vi "FlatToRichw4lvgrpc_Msg_ToClient_3.vi"(5 "OutputClusterType":T1, 11 "InputCluster":T3) -> (3 "OutputCluster":T1)   [LabVIEW 2019, in "Generated_server.lvlib"]
uses:
  Generated_server.lvlib
  w4lvgrpc_State.ctl
  w4lvgrpc_Msg_ToClient_3.ctl
  w4lvgrpc_Msg_ToClient_3_Flat.ctl
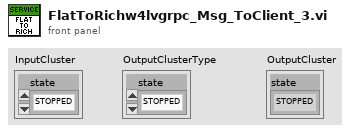
[diagram p1: front panel]
types:
  T1 = typedef "Generated_server.lvlib/w4lvgrpc_Msg_ToClient_3.ctl" = cluster{"state":T2}
  T2 = typedef "Generated_server.lvlib/w4lvgrpc_State.ctl" = enum32{"STOPPED", "RUNNING", "ERROR"}
  T3 = typedef "Generated_server.lvlib/w4lvgrpc_Msg_ToClient_3_Flat.ctl" = cluster{"state":T2}
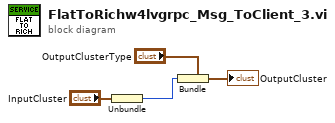
[diagram p0: block diagram]
diagram:
  n1 = Unbundle "Unbundle"("InputCluster") -> ("state"=w1:T2)
  n2 = Bundle "Bundle"(cluster="OutputClusterType", "state"=w1) -> (→"OutputCluster":T1)
